vi "create_folder_recursive.vi"(8 "error in":errorcluster, 11 "path in":path) -> (0 "error out":errorcluster, 3 "path out":path)   [LabVIEW 2015, in "lv-config-json-indexable.lvlib"]
uses:
  lv-config-json-indexable.lvlib
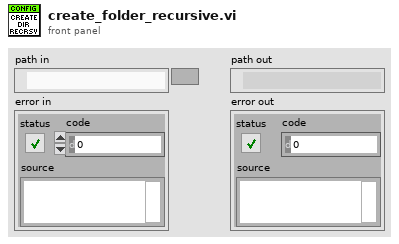
[diagram p1: front panel]
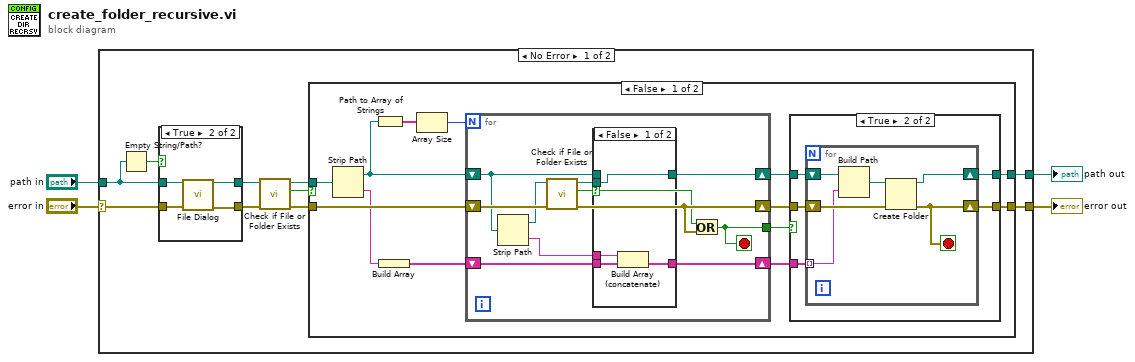
[diagram p0: block diagram]
diagram:
  n1 = case shown="No Error" "error in" {
    selector: "error in" -> [w12 w65]
    tunnel: "path in" -> [w14 _]
    tunnel: [w6 w65] -> w3
    tunnel: [w5 _] -> w4
    frame No Error {
      n2 = Empty String/Path?(string/path=w14) -> (empty?=w13:bool)
      n3 = case shown="True" w13 {
        tunnel: w14 -> [w60 w64]
        tunnel: [w60 w63] -> w11
        tunnel: w12 -> [w59 w62]
        tunnel: [w59 w61] -> w10
        frame False {
        }
        frame True {
          n4 = call "File Dialog"("start path"=w64, "error in"=w62) -> ("selected path"=w63:path, "error out"=w61:errorcluster)  [unwired: 10 in, 2 out]
        }
      }
      n5 = call <vilib>:"Check if File or Folder Exists.vi"("error in (no error)"=w10, "path"=w11) -> ("error out"=w8:errorcluster, "file or folder exists?"=w7:bool, "dup path"=w9:path)  [unwired: 7 in]
      n6 = case shown="False" w7 {
        tunnel: w9 -> [w24 w57]
        tunnel: w8 -> [w25 w58]
        tunnel: [w17 w58] -> w6
        tunnel: [w16 w57] -> w5
        frame False {
          n7 = Strip Path(path=w24) -> (stripped path=w21:path, name=w23:string)
          n8 = Path to Array of Strings(0:w21) -> (2:w27:string[])  [unwired: 1 out]
          n9 = Build Array(w23) -> (w22:string[])
          n10 = Array Size(array=w27) -> (size(s)=w26:i32)
          n11 = for {
            N: w26 -> [_]
            shift-right: [w29] -> w19
            shift-left: w21 -> [w31]
            shift-right: [w37] -> w18
            shift-left: w25 -> [w38]
            tunnel: [w35] -> w20
            shift-right: [w34] -> w15
            shift-left: w22 -> [w33]
            stop <- w35 stop-if-true
            n12 = Strip Path(path=w31) -> (stripped path=w36:path, name=w32:string)
            n13 = call <vilib>:"Check if File or Folder Exists.vi"("error in (no error)"=w38, "path"=w36) -> ("error out"=w37:errorcluster, "file or folder exists?"=w28:bool, "dup path"=w30:path)  [unwired: 7 in]
            n14 = case shown="False" w28 {
              tunnel: [w42 w43] -> w34
              tunnel: w33 -> [w41 w43]
              tunnel: w32 -> [w40 _]
              tunnel: w31 -> [_ w44]
              tunnel: w30 -> [w39 _]
              tunnel: [w39 w44] -> w29
              frame False {
                n15 = Build Array (concatenate)(w40, w41) -> (w42:string[])
              }
              frame True {
              }
            }
            n16 = Or(x=w28, y=w37) -> (x .or. y?=w35:bool)
          }
          n17 = case shown="True" w20 {
            tunnel: w19 -> [_ w49]
            tunnel: w18 -> [w45 w48]
            tunnel: w15 -> [_ w50]
            tunnel: [w45 w46] -> w17
            tunnel: [_ w47] -> w16
            frame False {
            }
            frame True {
              n18 = for {
                tunnel: w50 -> [w54] mode=indexing
                shift-right: [w51] -> w47
                shift-left: w49 -> [w55]
                shift-right: [w52] -> w46
                shift-left: w48 -> [w56]
                stop <- w52 stop-if-true
                n19 = Build Path(base path=w55, name or relative path=w54) -> (appended path=w53:path)
                n20 = Create Folder(path (use dialog)=w53, error in=w56) -> (created path=w51:path, error out=w52:errorcluster)  [unwired: 1 in, 1 out]
              }
            }
          }
        }
        frame True {
        }
      }
    }
    frame Error {
    }
  }
  "error out" <- w3
  "path out" <- w4
